vi "Read WebSocket Options.vi"(8 "error in (no error)":errorcluster, 11 "WAMP Client in":refnum<class "WAMP Client.lvclass">) -> (0 "error out":errorcluster, 2 "WebSocket Options":T1, 3 "WAMP Client out":refnum<class "WAMP Client.lvclass">)   [LabVIEW 2020, in "wamplv.lvlib" / "WAMP Client.lvclass"]
uses:
  WAMP Client.lvclass
  Private/Comm Handlers/Websocket Handler/Options.ctl
  Private/Comm Handlers/Websocket Handler/Headers.ctl
  WAMP Client.lvclass/WAMP Client.ctl
  Private/Comm Handlers/Websocket Handler/Websocket Handler.lvclass
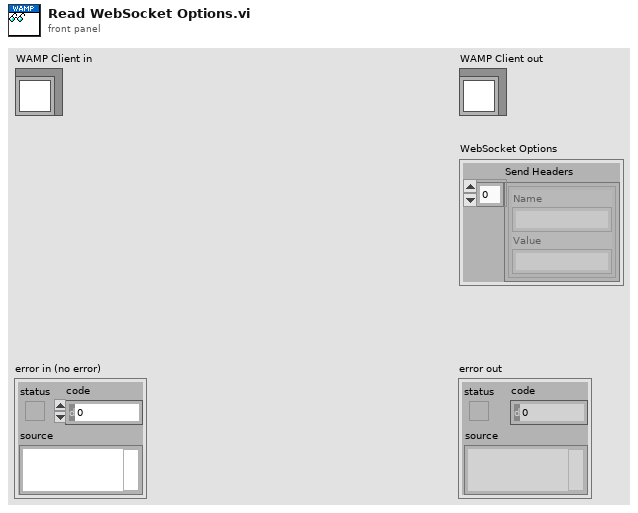
[diagram p1: front panel]
types:
  T1 = typedef "wamplv.lvlib/Websocket Handler.lvclass/Options.ctl" = cluster{"Send Headers":T2[]}
  T2 = typedef "wamplv.lvlib/Websocket Handler.lvclass/Headers.ctl" = cluster{"Name":string, "Value":string}
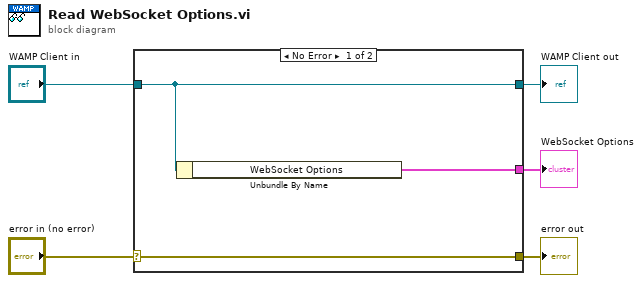
[diagram p0: block diagram]
diagram:
  n1 = case shown="No Error" "error in (no error)" {
    selector: "error in (no error)" -> [w8 w9]
    tunnel: [w8 w9] -> w4
    tunnel: [w7 w10] -> w2
    tunnel: "WAMP Client in" -> [w7 w10]
    tunnel: [w6 _] -> w1
    frame No Error {
      n2 = Unbundle By Name(w7) -> ("WebSocket Options"=w6:T1)
    }
    frame Error {
    }
  }
  "error out" <- w4
  "WAMP Client out" <- w2
  "WebSocket Options" <- w1
